vi "Read New Panel UE.vi"(8 "error in (no error)":errorcluster, 11 "TipPanel in":refnum<class "TipPanel.lvclass">) -> (0 "error out":errorcluster, 2 "UE: ToPanel":refnum<user-event>, 3 "TipPanel out":refnum<class "TipPanel.lvclass">)   [LabVIEW 2021, in "TipStripOOPanel.lvlib" / "TipPanel.lvclass"]
uses:
  TipPanel.lvclass
  ToPanelUEWrapper.ctl
  ToPanelUE.ctl
  <vilib>/Futures/Futures/Promise/Promise.lvclass
  TipPanel.lvclass/TipPanel.ctl
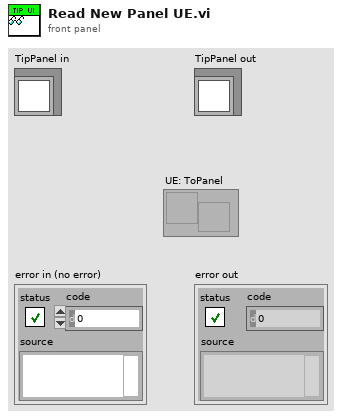
[diagram p1: front panel]
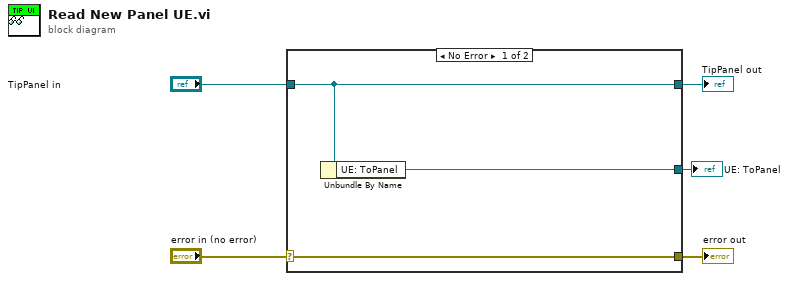
[diagram p0: block diagram]
diagram:
  n1 = case shown="No Error" "error in (no error)" {
    selector: "error in (no error)" -> [w8 w9]
    tunnel: [w8 w9] -> w4
    tunnel: [w7 w10] -> w2
    tunnel: "TipPanel in" -> [w7 w10]
    tunnel: [w6 _] -> w1
    frame No Error {
      n2 = Unbundle By Name(w7) -> ("UE: ToPanel"=w6:refnum<user-event>)
    }
    frame Error {
    }
  }
  "error out" <- w4
  "TipPanel out" <- w2
  "UE: ToPanel" <- w1
